vi "Finalize.vi"(8 "error in (no error)":errorcluster, 11 "ADAS PE Template in":refnum<class "ADAS PE Template.lvclass">) -> (0 "error out":errorcluster, 3 "ADAS PE Template out":refnum<class "ADAS PE Template.lvclass">)   [LabVIEW 2020, in "ADAS PE Template.lvlib" / "ADAS PE Template.lvclass"]
doc: "<b>Finalize</b>\nThis method is called as the plugin is shut down. If there are any short-duration post-processing actions (such as writing a summary/index file of data just recorded by the plugin) or lifetime references (like DVRs of shared data used with the Handle Message method), make sure to finalize those here."
uses:
  ADAS PE Template.lvclass
  C:/Program Files/National Instruments/LabVIEW 2020/vi.lib/FlexLogger/SDK/PluginSDK.lvlibp/PEFClasses/SDK/Processing Element/Processing Element.lvclass
  <vilib>/FlexLogger/SDK/PluginSDK.lvlibp/PEFClasses/SDK/Processing Element/Read Alias.vi
  <vilib>/ADAS Record/Tracing/GenericEventStart.vi
  <vilib>/ADAS Record/Tracing/GenericEventStop.vi
  <vilib>/ADAS Record/Utilities/ADAS Utilities.lvlib
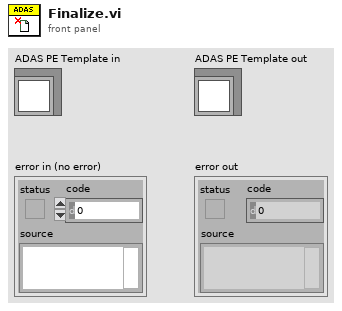
[diagram p1: front panel]
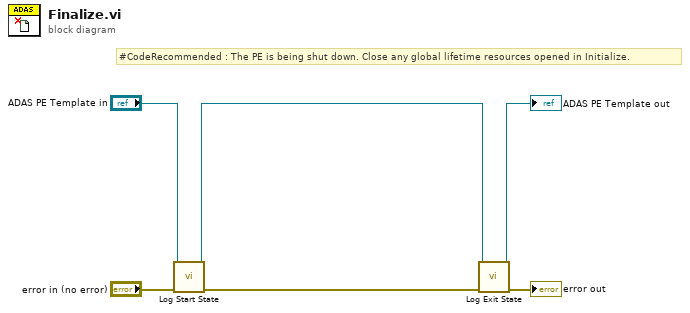
[diagram p0: block diagram]
diagram:
  # "#CodeRecommended : The PE is being shut down. Close any global lifetime resources opened in Initialize."
  n1 = call <vilib>:"Log Start State.vi"("error in (no error)"="error in (no error)", "PluginSDK.lvlibp:Processing Element.lvclass"="ADAS PE Template in") -> ("error out"=w5:errorcluster, "PluginSDK.lvlibp:Processing Element.lvclass"=w2:refnum<class "ADAS PE Template.lvclass">)  [unwired: 8 in]
  n2 = call <vilib>:"Log Exit State.vi"("error in (no error)"=w5, "PluginSDK.lvlibp:Processing Element.lvclass"=w2) -> ("error out"=→"error out":errorcluster, "PluginSDK.lvlibp:Processing Element.lvclass"=→"ADAS PE Template out":refnum<class "ADAS PE Template.lvclass">)  [unwired: 8 in]
